vi "MGCC_PVFcst_PF.vi"(1 "InputTimeSeries":dbl[](array[numeric])) -> (0 "predicted series":dbl[](array[numeric]) format="%.4f")   [LabVIEW 2016]
doc: "This VI implements an ARMA model for time-series data forecasting."
uses:
  <vilib>/addons/Time Series Analysis/Modeling and Prediction.llb/TSA AR Modeling Order (Array).vi
  <vilib>/addons/Time Series Analysis/Modeling and Prediction.llb/TSA ARMA Modeling (Array).vi
  <vilib>/addons/Time Series Analysis/Modeling and Prediction.llb/TSA ARMA Prediction (Array).vi
  <vilib>/addons/_Advanced Signal Processing/NI_AdvSigProcTSA.lvlib
panel:
  out "standard deviation":dbl[](array[numeric]) format="%.4f"
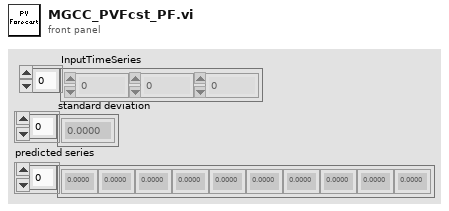
[diagram p1: front panel]
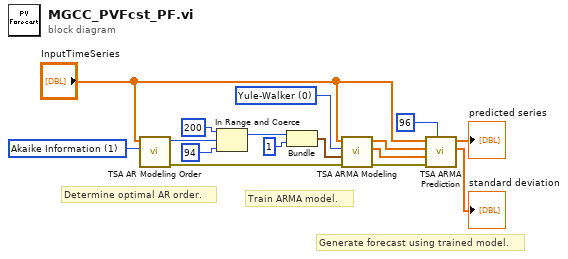
[diagram p0: block diagram]
diagram:
  w9 = 1 items=["Final Prediction Error"=0, "Akaike Information"=1, "Bayesian Information"=4, "Minimal Description Length"=2, "Phi Criterion"=3, "-"=-1, "Partial Correlation Function"=6] ("method")
  w10 = u16 0 items=["Yule-Walker", "High order AR", "Polynomial"] ("method")
  # "Generate forecast using trained model."
  # "Train ARMA model."
  # "Determine optimal AR order."
  n1 = call-poly <vilib>:"TSA AR Modeling Order.vi"("method"=w9, "Xt"="InputTimeSeries") -> ("error out"=w7:errorcluster, "optimal AR order"=w5:i32)  [unwired: 7 in, 1 out]
  n2 = In Range and Coerce(upper limit=200, x=w5, lower limit=94) -> (coerced(x)=w3:i32)  [unwired: 1 out]
  n3 = Bundle("upper limit"=w3, 1) -> (w1:cluster{"upper limit":i32, i32})  [unwired: 1 in]
  n4 = call-poly <vilib>:"TSA ARMA Modeling.vi"("error in (no error)"=w7, "ARMA order"=w1, "method"=w10, "Xt"="InputTimeSeries") -> ("error out"=w14:errorcluster, "MA coefficients"=w12:dbl[], "AR coefficients"=w13:dbl[])  [unwired: 4 in, 1 out]
  n5 = call-poly <vilib>:"TSA ARMA Prediction.vi"("number of points"=96, "error in (no error)"=w14, "MA coefficients"=w12, "AR coefficients"=w13, "Xt"="InputTimeSeries") -> ("standard deviation"=→"standard deviation":dbl[], "predicted series"=→"predicted series":dbl[])  [unwired: 4 in, 1 out]
